vi "Initiate Updates.vi"(8 "error in (no error)":errorcluster, 11 "IDialogBox In":refnum<class "IDialogBox.lvclass">) -> (0 "error out":errorcluster, 3 "IDialogBox Out":refnum<class "IDialogBox.lvclass">)   [LabVIEW 2017, in "IDialogBox.lvlib" / "IDialogBox.lvclass"]
doc: "<License>\nCopyright © 2017 Composed Systems, LLC | All rights reserved\nwww.composed.io\n\nAuthor: Ethan Stern <ethan.stern@composed.io>\n\nThis software is provided \"AS IS\" WITHOUT WARRANTIES, either express or implied, AND IS FOR EDUCATIONAL PURPOSES ONLY.\n</License>"
uses:
  IDialogBox.lvclass
  C:/Git/mva-framework/Framework/IViewable/IViewable/IViewable.lvclass
  IViewable/IViewable/IViewable.lvclass/IViewable.ctl
  IViewable/IViewable/IViewable.lvclass
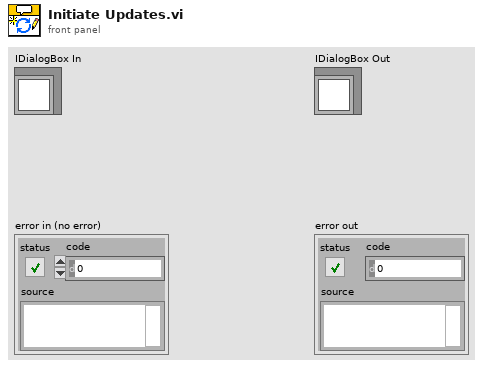
[diagram p1: front panel]
types:
  T1 = enum32{"Invalid", "Standard", "Closed", "Hidden", "Minimized", "Maximized"}
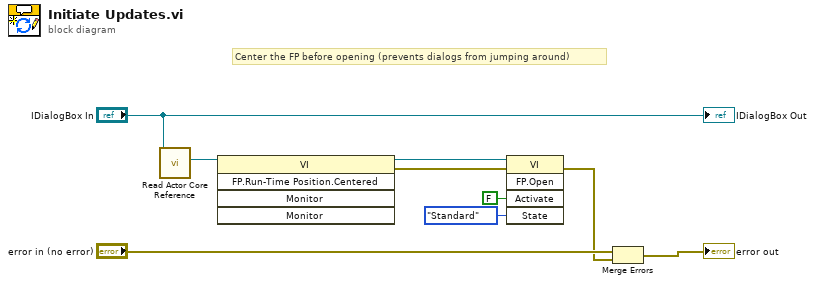
[diagram p0: block diagram]
diagram:
  # "Center the FP before opening (prevents dialogs from jumping around)"
  n1 = call "Read Actor Core Reference.vi"("IViewable In"="IDialogBox In") -> ("Actor Core Refnum"=w1:refnum<vi>)  [unwired: 9 in, 1 out]
  n2 = invoke class="VI" method="FP.Run-Time Position.Centered"(reference=w1) -> (reference out=w4:refnum<vi>, error out=w6:errorcluster)  [unwired: 4 in, 3 out]
  n3 = invoke class="VI" method="FP.Open"(reference=w4, error in=w6, "Activate"=FALSE ("Activate?"), "State"=T1."Standard") -> (error out=w5:errorcluster)  [unwired: 1 in, 4 out]
  n4 = Merge Errors("error in (no error)", w5) -> (→"error out":errorcluster)
  "IDialogBox Out" <- "IDialogBox In"
